vi "set lights for given state BAP4B.vi"(7 "light state":T1) -> (8 "all lights out":T2)   [LabVIEW 2014]
doc: "This vi sets the particular light on/off configuration for all of the lights in the intersection state machine appropriate to a particular state.\n\nPaul K Dixon\nP350\nCSUSB Physics"
uses:
  typedefs/all lights.ctl
  typedefs/light set.ctl
  typedefs/stop light.ctl
  typedefs/left arrow.ctl
  typedefs/walk light.ctl
  typedefs/state enum.ctl
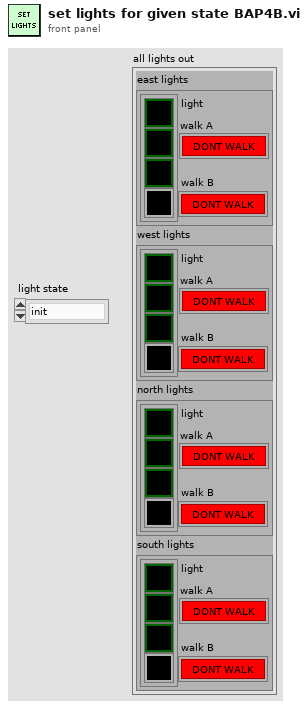
[diagram p1: front panel]
types:
  T1 = typedef "state enum.ctl" = enum16{"init", "idle", "left turn E", "go EW", "caution EW", "left turn W", "left turn N", "go NS", "caution NS", "left turn S", "blink on", "blink off", "all on test", "exit"}
  T2 = typedef "all lights.ctl" = cluster{"east lights":T3, "west lights":T3, "north lights":T3, "south lights":T3}
  T3 = typedef "light set.ctl" = cluster{"light":T4, "walk A":T6, "walk B":T6}
  T4 = typedef "stop light.ctl" = cluster{"stop":bool, "caution":bool, "go":bool, "arrow":T5}
  T5 = typedef "left arrow.ctl" = bool
  T6 = typedef "walk light.ctl" = bool
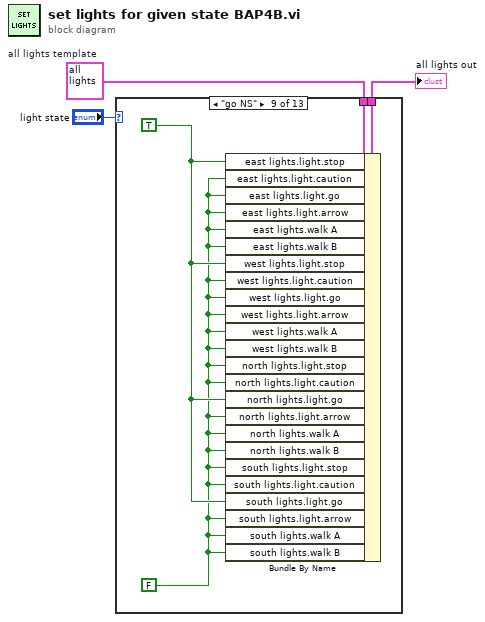
[diagram p0: block diagram]
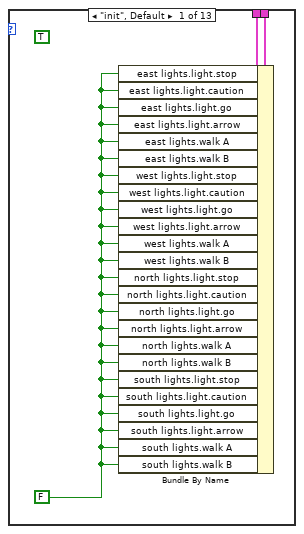
[diagram p2: hidden frame]
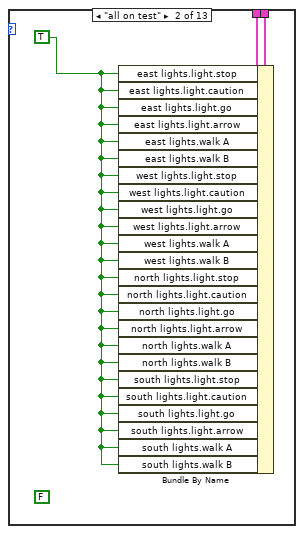
[diagram p3: hidden frame]
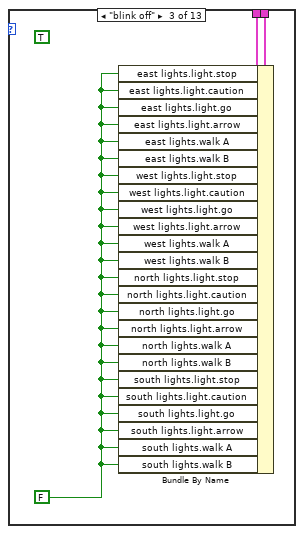
[diagram p4: hidden frame]
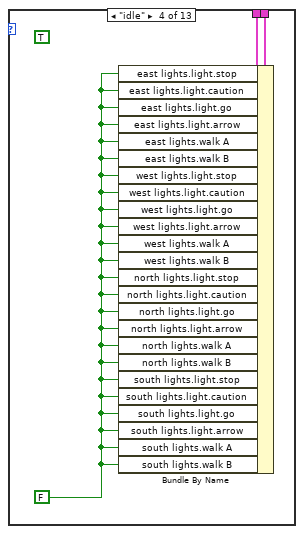
[diagram p5: hidden frame]
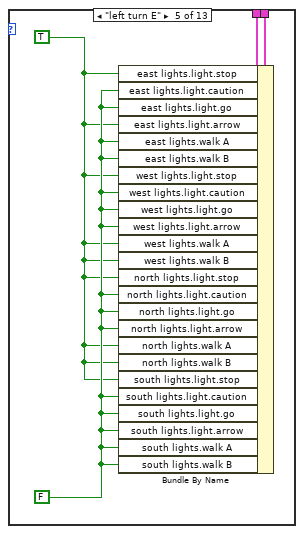
[diagram p6: hidden frame]
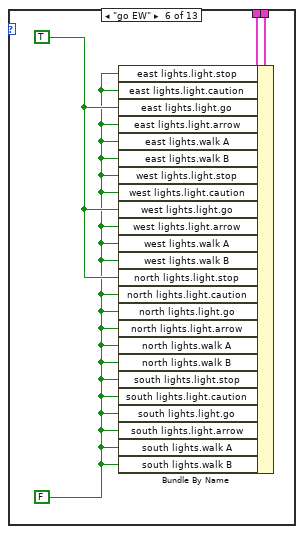
[diagram p7: hidden frame]
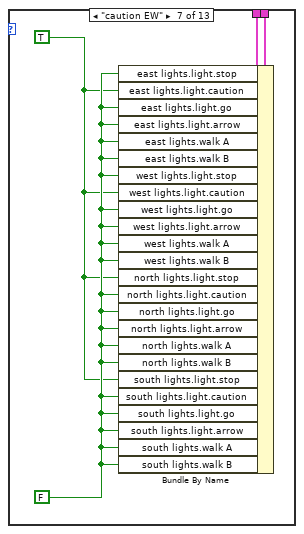
[diagram p8: hidden frame]
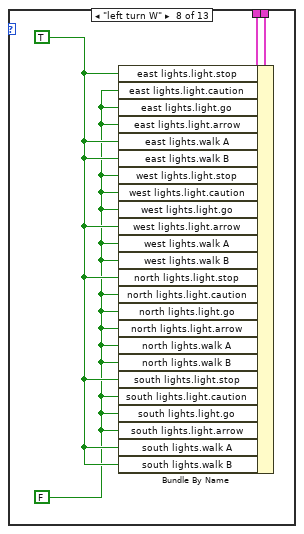
[diagram p9: hidden frame]
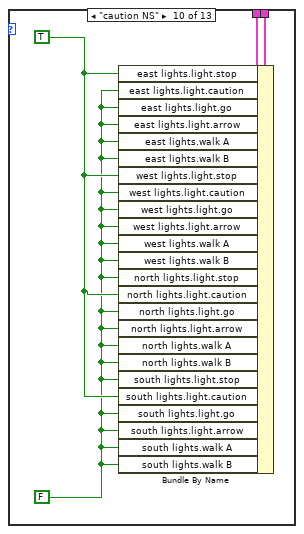
[diagram p10: hidden frame]
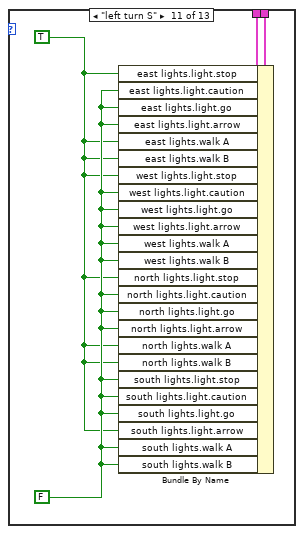
[diagram p11: hidden frame]
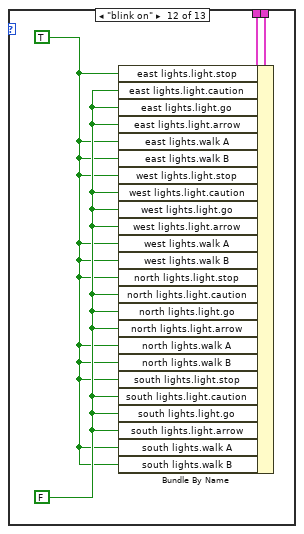
[diagram p12: hidden frame]
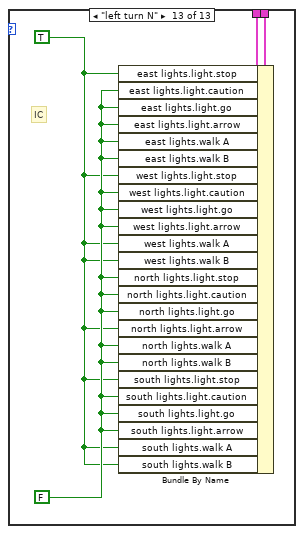
[diagram p13: hidden frame]
diagram:
  w2 = T2 {"east lights"={"light"={"stop"=FALSE, "caution"=FALSE, "go"=FALSE, "arrow"=FALSE}, "walk A"=FALSE, "walk B"=FALSE}, "west lights"={"light"={"stop"=FALSE, "caution"=FALSE, "go"=FALSE, "arrow"=FALSE}, "walk A"=FALSE, "walk B"=FALSE}, "north lights"={"light"={"stop"=FALSE, "caution"=FALSE, "go"=FALSE, "arrow"=FALSE}, "walk A"=FALSE, "walk B"=FALSE}, "south lights"={"light"={"stop"=FALSE, "caution"=FALSE, "go"=FALSE, "arrow"=FALSE}, "walk A"=FALSE, "walk B"=FALSE}}  # all lights template
  n1 = case shown="\"go NS\"" "light state" {
    tunnel: w2 -> [w6 w9 w12 w15 w19 w23 w27 w31 w35 w39 w43 w47 w51]
    tunnel: [w5 w8 w11 w14 w18 w22 w26 w30 w34 w38 w42 w46 w50] -> w1
    frame "init", Default {
      (unwired) TRUE
      w4 = FALSE
      n2 = Bundle By Name(cluster=w6, "east lights.light.stop"=w4, "east lights.light.caution"=w4, "east lights.light.go"=w4, "east lights.light.arrow"=w4, "east lights.walk A"=w4, "east lights.walk B"=w4, "west lights.light.stop"=w4, "west lights.light.caution"=w4, "west lights.light.go"=w4, "west lights.light.arrow"=w4, "west lights.walk A"=w4, "west lights.walk B"=w4, "north lights.light.stop"=w4, "north lights.light.caution"=w4, "north lights.light.go"=w4, "north lights.light.arrow"=w4, "north lights.walk A"=w4, "north lights.walk B"=w4, "south lights.light.stop"=w4, "south lights.light.caution"=w4, "south lights.light.go"=w4, "south lights.light.arrow"=w4, "south lights.walk A"=w4, "south lights.walk B"=w4) -> (w5:T2)
    }
    frame "all on test" {
      w7 = TRUE
      (unwired) FALSE
      n3 = Bundle By Name(cluster=w9, "east lights.light.stop"=w7, "east lights.light.caution"=w7, "east lights.light.go"=w7, "east lights.light.arrow"=w7, "east lights.walk A"=w7, "east lights.walk B"=w7, "west lights.light.stop"=w7, "west lights.light.caution"=w7, "west lights.light.go"=w7, "west lights.light.arrow"=w7, "west lights.walk A"=w7, "west lights.walk B"=w7, "north lights.light.stop"=w7, "north lights.light.caution"=w7, "north lights.light.go"=w7, "north lights.light.arrow"=w7, "north lights.walk A"=w7, "north lights.walk B"=w7, "south lights.light.stop"=w7, "south lights.light.caution"=w7, "south lights.light.go"=w7, "south lights.light.arrow"=w7, "south lights.walk A"=w7, "south lights.walk B"=w7) -> (w8:T2)
    }
    frame "blink off" {
      (unwired) TRUE
      w10 = FALSE
      n4 = Bundle By Name(cluster=w12, "east lights.light.stop"=w10, "east lights.light.caution"=w10, "east lights.light.go"=w10, "east lights.light.arrow"=w10, "east lights.walk A"=w10, "east lights.walk B"=w10, "west lights.light.stop"=w10, "west lights.light.caution"=w10, "west lights.light.go"=w10, "west lights.light.arrow"=w10, "west lights.walk A"=w10, "west lights.walk B"=w10, "north lights.light.stop"=w10, "north lights.light.caution"=w10, "north lights.light.go"=w10, "north lights.light.arrow"=w10, "north lights.walk A"=w10, "north lights.walk B"=w10, "south lights.light.stop"=w10, "south lights.light.caution"=w10, "south lights.light.go"=w10, "south lights.light.arrow"=w10, "south lights.walk A"=w10, "south lights.walk B"=w10) -> (w11:T2)
    }
    frame "idle" {
      (unwired) TRUE
      w13 = FALSE
      n5 = Bundle By Name(cluster=w15, "east lights.light.stop"=w13, "east lights.light.caution"=w13, "east lights.light.go"=w13, "east lights.light.arrow"=w13, "east lights.walk A"=w13, "east lights.walk B"=w13, "west lights.light.stop"=w13, "west lights.light.caution"=w13, "west lights.light.go"=w13, "west lights.light.arrow"=w13, "west lights.walk A"=w13, "west lights.walk B"=w13, "north lights.light.stop"=w13, "north lights.light.caution"=w13, "north lights.light.go"=w13, "north lights.light.arrow"=w13, "north lights.walk A"=w13, "north lights.walk B"=w13, "south lights.light.stop"=w13, "south lights.light.caution"=w13, "south lights.light.go"=w13, "south lights.light.arrow"=w13, "south lights.walk A"=w13, "south lights.walk B"=w13) -> (w14:T2)
    }
    frame "left turn E" {
      w16 = TRUE
      w17 = FALSE
      n6 = Bundle By Name(cluster=w19, "east lights.light.stop"=w16, "east lights.light.caution"=w17, "east lights.light.go"=w17, "east lights.light.arrow"=w16, "east lights.walk A"=w17, "east lights.walk B"=w17, "west lights.light.stop"=w16, "west lights.light.caution"=w17, "west lights.light.go"=w17, "west lights.light.arrow"=w17, "west lights.walk A"=w16, "west lights.walk B"=w16, "north lights.light.stop"=w16, "north lights.light.caution"=w17, "north lights.light.go"=w17, "north lights.light.arrow"=w17, "north lights.walk A"=w16, "north lights.walk B"=w16, "south lights.light.stop"=w16, "south lights.light.caution"=w17, "south lights.light.go"=w17, "south lights.light.arrow"=w17, "south lights.walk A"=w17, "south lights.walk B"=w17) -> (w18:T2)
    }
    frame "go EW" {
      w21 = TRUE
      w20 = FALSE
      n7 = Bundle By Name(cluster=w23, "east lights.light.stop"=w20, "east lights.light.caution"=w20, "east lights.light.go"=w21, "east lights.light.arrow"=w20, "east lights.walk A"=w20, "east lights.walk B"=w20, "west lights.light.stop"=w20, "west lights.light.caution"=w20, "west lights.light.go"=w21, "west lights.light.arrow"=w20, "west lights.walk A"=w20, "west lights.walk B"=w20, "north lights.light.stop"=w21, "north lights.light.caution"=w20, "north lights.light.go"=w20, "north lights.light.arrow"=w20, "north lights.walk A"=w20, "north lights.walk B"=w20, "south lights.light.stop"=w20, "south lights.light.caution"=w20, "south lights.light.go"=w20, "south lights.light.arrow"=w20, "south lights.walk A"=w20, "south lights.walk B"=w20) -> (w22:T2)
    }
    frame "caution EW" {
      w24 = TRUE
      w25 = FALSE
      n8 = Bundle By Name(cluster=w27, "east lights.light.stop"=w25, "east lights.light.caution"=w24, "east lights.light.go"=w25, "east lights.light.arrow"=w25, "east lights.walk A"=w25, "east lights.walk B"=w25, "west lights.light.stop"=w25, "west lights.light.caution"=w24, "west lights.light.go"=w25, "west lights.light.arrow"=w25, "west lights.walk A"=w25, "west lights.walk B"=w25, "north lights.light.stop"=w24, "north lights.light.caution"=w25, "north lights.light.go"=w25, "north lights.light.arrow"=w25, "north lights.walk A"=w25, "north lights.walk B"=w25, "south lights.light.stop"=w24, "south lights.light.caution"=w25, "south lights.light.go"=w25, "south lights.light.arrow"=w25, "south lights.walk A"=w25, "south lights.walk B"=w25) -> (w26:T2)
    }
    frame "left turn W" {
      w29 = TRUE
      w28 = FALSE
      n9 = Bundle By Name(cluster=w31, "east lights.light.stop"=w29, "east lights.light.caution"=w28, "east lights.light.go"=w28, "east lights.light.arrow"=w28, "east lights.walk A"=w29, "east lights.walk B"=w29, "west lights.light.stop"=w28, "west lights.light.caution"=w28, "west lights.light.go"=w28, "west lights.light.arrow"=w29, "west lights.walk A"=w28, "west lights.walk B"=w28, "north lights.light.stop"=w29, "north lights.light.caution"=w28, "north lights.light.go"=w28, "north lights.light.arrow"=w28, "north lights.walk A"=w28, "north lights.walk B"=w28, "south lights.light.stop"=w29, "south lights.light.caution"=w28, "south lights.light.go"=w28, "south lights.light.arrow"=w28, "south lights.walk A"=w29, "south lights.walk B"=w29) -> (w30:T2)
    }
    frame "go NS" {
      w33 = TRUE
      w32 = FALSE
      n10 = Bundle By Name(cluster=w35, "east lights.light.stop"=w33, "east lights.light.caution"=w32, "east lights.light.go"=w32, "east lights.light.arrow"=w32, "east lights.walk A"=w32, "east lights.walk B"=w32, "west lights.light.stop"=w33, "west lights.light.caution"=w32, "west lights.light.go"=w32, "west lights.light.arrow"=w32, "west lights.walk A"=w32, "west lights.walk B"=w32, "north lights.light.stop"=w32, "north lights.light.caution"=w32, "north lights.light.go"=w33, "north lights.light.arrow"=w32, "north lights.walk A"=w32, "north lights.walk B"=w32, "south lights.light.stop"=w32, "south lights.light.caution"=w32, "south lights.light.go"=w33, "south lights.light.arrow"=w32, "south lights.walk A"=w32, "south lights.walk B"=w32) -> (w34:T2)
    }
    frame "caution NS" {
      w37 = TRUE
      w36 = FALSE
      n11 = Bundle By Name(cluster=w39, "east lights.light.stop"=w37, "east lights.light.caution"=w36, "east lights.light.go"=w36, "east lights.light.arrow"=w36, "east lights.walk A"=w36, "east lights.walk B"=w36, "west lights.light.stop"=w37, "west lights.light.caution"=w36, "west lights.light.go"=w36, "west lights.light.arrow"=w36, "west lights.walk A"=w36, "west lights.walk B"=w36, "north lights.light.stop"=w36, "north lights.light.caution"=w37, "north lights.light.go"=w36, "north lights.light.arrow"=w36, "north lights.walk A"=w36, "north lights.walk B"=w36, "south lights.light.stop"=w36, "south lights.light.caution"=w37, "south lights.light.go"=w36, "south lights.light.arrow"=w36, "south lights.walk A"=w36, "south lights.walk B"=w36) -> (w38:T2)
    }
    frame "left turn S" {
      w40 = TRUE
      w41 = FALSE
      n12 = Bundle By Name(cluster=w43, "east lights.light.stop"=w40, "east lights.light.caution"=w41, "east lights.light.go"=w41, "east lights.light.arrow"=w41, "east lights.walk A"=w40, "east lights.walk B"=w40, "west lights.light.stop"=w40, "west lights.light.caution"=w41, "west lights.light.go"=w41, "west lights.light.arrow"=w41, "west lights.walk A"=w41, "west lights.walk B"=w41, "north lights.light.stop"=w40, "north lights.light.caution"=w41, "north lights.light.go"=w41, "north lights.light.arrow"=w41, "north lights.walk A"=w40, "north lights.walk B"=w40, "south lights.light.stop"=w41, "south lights.light.caution"=w41, "south lights.light.go"=w41, "south lights.light.arrow"=w40, "south lights.walk A"=w41, "south lights.walk B"=w41) -> (w42:T2)
    }
    frame "blink on" {
      w44 = TRUE
      w45 = FALSE
      n13 = Bundle By Name(cluster=w47, "east lights.light.stop"=w44, "east lights.light.caution"=w45, "east lights.light.go"=w45, "east lights.light.arrow"=w45, "east lights.walk A"=w44, "east lights.walk B"=w44, "west lights.light.stop"=w44, "west lights.light.caution"=w45, "west lights.light.go"=w45, "west lights.light.arrow"=w45, "west lights.walk A"=w44, "west lights.walk B"=w44, "north lights.light.stop"=w44, "north lights.light.caution"=w45, "north lights.light.go"=w45, "north lights.light.arrow"=w45, "north lights.walk A"=w44, "north lights.walk B"=w44, "south lights.light.stop"=w44, "south lights.light.caution"=w45, "south lights.light.go"=w45, "south lights.light.arrow"=w45, "south lights.walk A"=w44, "south lights.walk B"=w44) -> (w46:T2)
    }
    frame "left turn N" {
      w48 = TRUE
      w49 = FALSE
      # "IC"
      n14 = Bundle By Name(cluster=w51, "east lights.light.stop"=w48, "east lights.light.caution"=w49, "east lights.light.go"=w49, "east lights.light.arrow"=w49, "east lights.walk A"=w49, "east lights.walk B"=w49, "west lights.light.stop"=w48, "west lights.light.caution"=w49, "west lights.light.go"=w49, "west lights.light.arrow"=w49, "west lights.walk A"=w48, "west lights.walk B"=w48, "north lights.light.stop"=w49, "north lights.light.caution"=w49, "north lights.light.go"=w49, "north lights.light.arrow"=w48, "north lights.walk A"=w49, "north lights.walk B"=w49, "south lights.light.stop"=w48, "south lights.light.caution"=w49, "south lights.light.go"=w49, "south lights.light.arrow"=w49, "south lights.walk A"=w48, "south lights.walk B"=w48) -> (w50:T2)
    }
  }
  "all lights out" <- w1
